vi "U3 Quadrature.vi"(8 "error in":errorcluster) -> (0 "error out":errorcluster)   [LabVIEW 2021]
panel:
  in  "Iteration Interval [ms]":u32=1000
  out "Pulses/Second":dbl
  out "Counts/Second":i32
  in  "Stop":bool
  in  "Reset Count":bool
  out "Quadrature Count":i32
  in  "FirstFound":bool=TRUE
  in  "Address":string="1"
  out "Error Message":string
  # "Demonstrates 1 quadrature input, which uses two timer channels for phases A and B (FIO4 and FIO5 in this case).\nIf you don't have a quadrature signal source handy, you can connect wires to GND, and tap these wires on FIO4\nand FIO5 to simulate quadrature."
  # "This VI passes a timer\nbase clock constant that\nis valid for hardware V1.21.\nFor hardware V1.20 change\nLJ_tc48MHZ to LJ_tc24MHZ."
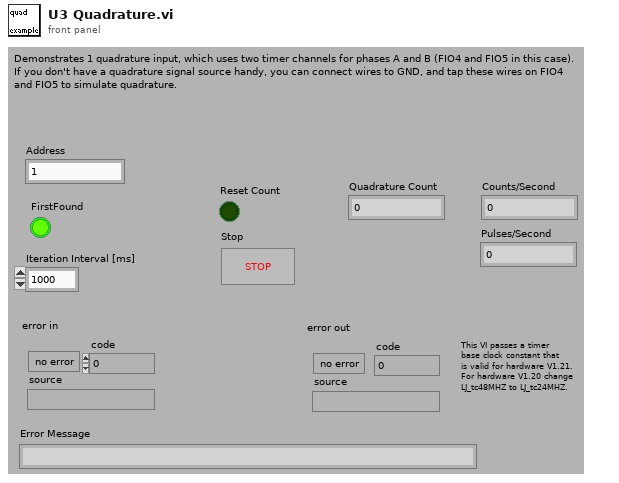
[diagram p1: front panel]
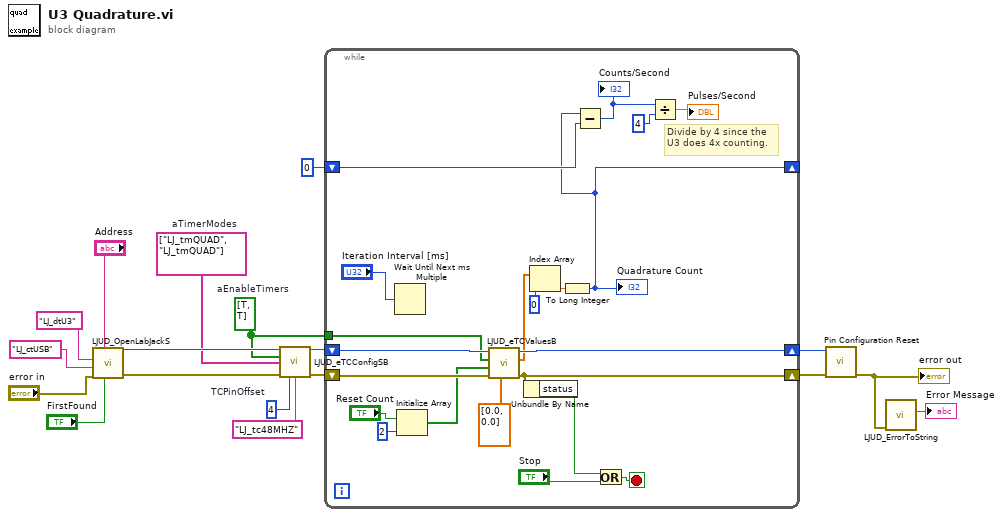
[diagram p0: block diagram]
diagram:
  w3 = 4  # TCPinOffset
  w2 = bool[] [TRUE, TRUE]  # aEnableTimers
  w5 = string[] ["LJ_tmQUAD", "LJ_tmQUAD"]  # aTimerModes
  n1 = call "LJUD_OpenLabJackS.vi"("FirstFound"="FirstFound", "Address"="Address", "error in"="error in", "ConnectionType"="LJ_ctUSB", "DeviceType"="LJ_dtU3") -> ("error out"=w9:errorcluster, "Handle"=w8:i32)  [unwired: 4 in, 1 out]
  n2 = call "LJUD_eTCConfigSB.vi"("Handle In"=w8, "aEnableTimers"=w2, "aTimerModes"=w5, "error in"=w9, "TCPinOffset"=w3, "TimerClockBase"="LJ_tc48MHZ") -> ("Handle Out"=w6:i32, "error out"=w7:errorcluster)  [unwired: 8 in]
  n3 = while {
    tunnel: w2 -> [w27]
    shift-left: w7 -> [w29]
    shift-right: [w38] -> w11
    shift-left: w6 -> [w30]
    shift-right: [w32] -> w12
    shift-right: [w19] -> _
    shift-left: 0 -> [w24]
    stop <- w37 stop-if-true
    # "Divide by 4 since the\nU3 does 4x counting."
    n4 = Wait Until Next ms Multiple(millisecond multiple="Iteration Interval [ms]") -> ()  [unwired: 1 out]
    n5 = Initialize Array("Reset Count", 2 ("Dimension Size")) -> (w26:bool[])
    n6 = call "LJUD_eTCValuesB.vi"("aTimerValues Write"=dbl[] [0.0, 0.0], "error in"=w29, "aUpdateResetTimers"=w26, "aReadTimers"=w27, "Handle In"=w30) -> ("error out"=w38:errorcluster, "aTimerValues Read"=w31:dbl[], "Handle Out"=w32:i32)  [unwired: 3 in, 1 out]
    n7 = Unbundle By Name(w38) -> ("status"=w36:bool)
    n8 = Index Array(array=w31, index=0 ("Index")) -> (element=w23:dbl)
    n9 = To Long Integer(number=w23) -> (32bit integer=w19:i32)
    "Quadrature Count" <- w19
    n10 = Subtract(x=w19, y=w24) -> (x-y=w22:i32)
    "Counts/Second" <- w22
    n11 = Or(x=w36, y="Stop") -> (x .or. y?=w37:bool)
    n12 = Divide(x=w22, y=4) -> (x/y=→"Pulses/Second":dbl)
  }
  n13 = call "Pin Configuration Reset.vi"("error in"=w11, "Handle In"=w12) -> ("error out"=w10:errorcluster)  [unwired: 8 in, 1 out]
  "error out" <- w10
  n14 = call "LJUD_ErrorToString.vi"("error in"=w10) -> ("String"=→"Error Message":string)  [unwired: 10 in]
